vi "GenesysPS.MeasureVoltage.vi"(0 "i ref in":refnum<vi>, 5 "error in (no error)":errorcluster) -> (14 "i ref out":refnum<vi>, 19 "error out":errorcluster)   [LabVIEW 2014, in "GenesysPS.lvlib"]
doc: "VI to read out the voltage over RS485.\n\nLicense Agreement for this software:\n\nCopyright (C)\nGesellschaft für Schwerionenforschung, GSI\nPlanckstr. 1\n64291 Darmstadt\nGermany\n\nContact: D.Beck@gsi.de \n\nThis program is free software; you can redistribute it and/or modify it under the terms of the GNU General Public License as published by the Free Software Foundation; either version 2 of the license, or (at your option) any later version.\n\nThis program is distributed in the hope that it will be useful, but WITHOUT ANY WARRANTY; without even the implied warranty of MERCHANTABILITY or FITNESS FOR A PARTICULAR PURPOSE. See the GNU General License for more details (http://www.gnu.org).\n\nGesellschaft für Schwerionenforschung, GSI\nPlanckstr. 1, 64291 Darmstadt, Germany\nFor all questions and ideas contact: M.Richter@gsi.de, H.Brand@gsi.de or D.Beck@gsi.de.\nLast update: 17-JUN-2004"
uses:
  GenesysPS.lvlib
  CSinstr.lib/GENser/GENserDriver.lvlib
  CSCore/CSApplicationBaseClasses/PSChannelBase/PSChannelBase.lvlib
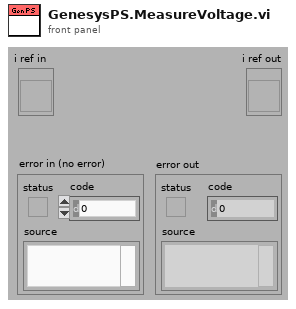
[diagram p1: front panel]
types:
  T1 = typedef "GenesysPS.lvlib/GenesysPS.i attribute.ctl" = cluster{"VISA name/ Heizinger":refnum<visa-resource-name>, "GEN Addr":i32, "WithTempInt?":bool, "TempLimit":dbl, "TemperatureID":i32, "Temp queue":refnum<queue>}
  T2 = typedef "PSChannelBase.lvlib/PSChannelBase.i attribute.ctl" = cluster{"defaultChannelIndex":i32, "nofChannels":i32, "defaultChannelIndexID":i32, "nofChannelsID":i32, "actValues":T3, "nomValues":T3, "logicalName":string[], "physicalName":string[], "logicalNameID":i32, "physicalNameID":i32}
  T3 = typedef "PSChannelBase.lvlib/PSChannelBase.parameters.ctl" = cluster{"onOff":bool[], "voltage":dbl[], "current":dbl[], "tripCurrent":dbl[], "rampUpSpeed":dbl[], "rampDownSpeed":dbl[], "status":i32[], "serviceIDs":cluster{"onOfflID":i32, "voltageID":i32, "currentID":i32, "tripCurrentID":i32, "rampUpSpeedID":i32, "rampDownSpeedID":i32, "statusID":i32}}
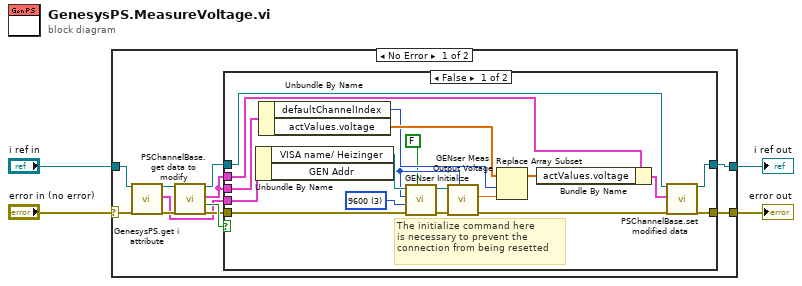
[diagram p0: block diagram]
diagram:
  n1 = case shown="No Error" "error in (no error)" {
    selector: "error in (no error)" -> [w9 w38]
    tunnel: [w13 w38] -> w4
    tunnel: [w12 w37] -> w2
    tunnel: "i ref in" -> [w8 w37]
    frame No Error {
      n2 = call "GenesysPS.get i attribute.vi"("i ref in"=w8, "error in (no error)"=w9) -> ("i ref out"=w7:refnum<vi>, "i attribute"=w6:T1, "error out"=w10:errorcluster)  [unwired: 15 in]
      n3 = call "PSChannelBase.get data to modify.vi"("i ref in"=w7, "error in (no error)"=w10) -> ("i ref out"=w11:refnum<vi>, "i attribute"=w5:T2, "timed out"=w15:bool, "error out"=w14:errorcluster)  [unwired: 14 in]
      n4 = case shown="False" w15 {
        tunnel: w11 -> [w31 w36]
        tunnel: w14 -> [w21 w35]
        tunnel: w6 -> [w34 _]
        tunnel: [w33 w35] -> w13
        tunnel: [w30 w36] -> w12
        tunnel: w5 -> [w29 _]
        tunnel: w5 -> [w27 _]
        frame False {
          w17 = u16 3 items=["1200", "2400", "4800", "9600", "19200"] ("BAUD")
          # "The initialize command here\nis necessary to prevent the\nconnection from being resetted"
          n5 = Unbundle By Name(w34) -> ("VISA name/ Heizinger"=w20:refnum<visa-resource-name>, "GEN Addr"=w18:i32)
          n6 = Unbundle By Name(w27) -> ("defaultChannelIndex"=w25:i32, "actValues.voltage"=w26:dbl[])
          n7 = call "GENser Initialize.vi"("Reset (T)"=FALSE, "error in (no error)"=w21, "BAUD"=w17, "GEN Addr"=w18, "VISA name"=w20) -> ("error out"=w22:errorcluster, "VISA out"=w19:refnum<visa-resource-name>)  [unwired: 5 in]
          n8 = call "GENser Meas Output Voltage.vi"("GEN Addr"=w18, "error"=w22, "VISA"=w19) -> ("error out"=w32:errorcluster, "Output Voltage"=w24:dbl)  [unwired: 6 in, 1 out]
          n9 = Replace Array Subset(array=w26, new element=w24, index=w25) -> (w23:dbl[])
          n10 = Bundle By Name(cluster=w29, "actValues.voltage"=w23) -> (w28:T2)
          n11 = call "PSChannelBase.set modified data.vi"("i ref in"=w31, "i attribute"=w28, "error in (no error)"=w32) -> ("i ref out"=w30:refnum<vi>, "error out"=w33:errorcluster)  [unwired: 15 in]
        }
        frame True {
        }
      }
    }
    frame Error {
    }
  }
  "i ref out" <- w2
  "error out" <- w4
